vi "Lab01_MyFirstVI.vi"() -> ()   [LabVIEW 2020]
panel:
  out "Status 1":bool
  in  "Switch 1":bool
  out "Status 2":bool
  in  "Switch 2":bool
  out "Status 3":bool
  in  "Switch 3":bool
  out "Indicator 4":dbl(knob) scale=0.0..10.0
  in  "Control 4":dbl(slide) scale=0.0..10.0
  out "Indicator 3":dbl(slide) scale=0.0..10.0 scale format="%#.3f"
  in  "Control 3":dbl(slide) scale=0.0..10.0 scale format="%#.3f"
  out "Indicator 2":dbl(slide) scale=0.0..100.0
  in  "Control 2":dbl(knob) scale=0.0..10.0 scale format="%#.2f"
  out "Indicator 1":dbl
  in  "Control 1":dbl
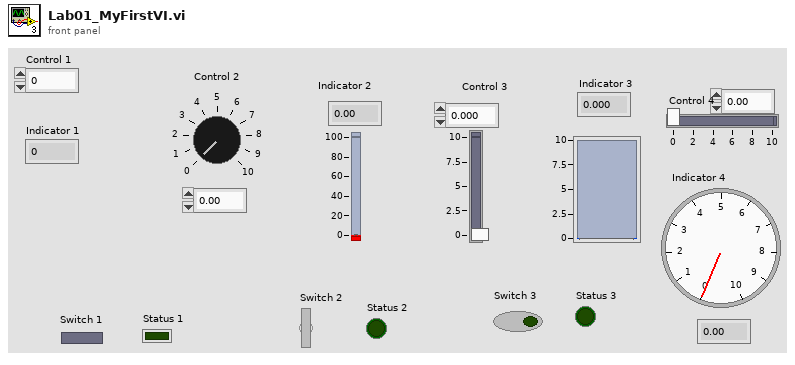
[diagram p1: front panel]
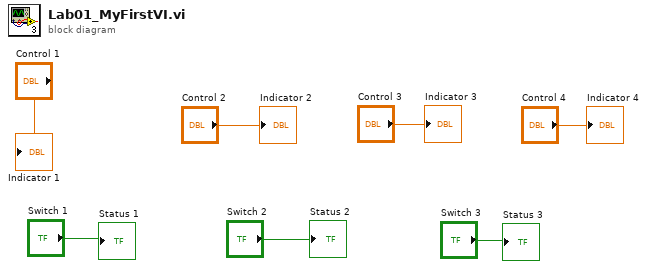
[diagram p0: block diagram]
diagram:
  "Indicator 1" <- "Control 1"
  "Indicator 2" <- "Control 2"
  "Indicator 3" <- "Control 3"
  "Indicator 4" <- "Control 4"
  "Status 3" <- "Switch 3"
  "Status 2" <- "Switch 2"
  "Status 1" <- "Switch 1"
